vi "End Array.vi"   [LabVIEW 2019, in "LabPack.lvlib" / "Reader.lvclass"]
doc: "Finishes reading an array from the MessagePack data. This must be called after reading all of the array elements."
uses:
  Reader.lvclass
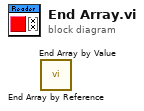
[diagram p0: block diagram]
diagram:
  n1 = call "End Array by Reference.vi"() -> ()  [unwired: 10 in, 2 out]
  n2 = call "End Array by Value.vi"() -> ()  [unwired: 10 in, 2 out]
